vi "UI Visible.vi"(8 "error in (no error)":errorcluster, 10 "UI visible?":bool, 11 "BluePlotHandle in":refnum<class "BluePlotHandle.lvclass">) -> (0 "error out":errorcluster, 3 "BluePlotHandle out":refnum<class "BluePlotHandle.lvclass">)   [LabVIEW 2021, in "BluePlot.lvlib" / "BluePlotHandle.lvclass"]
doc: "This is used to communicate to a plot instance whether or not it is visible.\n\nIf a plot instance is not visible, then it will not update to save performance.\n\nThis is necessary because the plot instance is not able to discern this information by itself"
uses:
  BluePlotHandle.lvclass
  BluePlotHandle.lvclass/BluePlotHandle.ctl
  TypeDefs/plot handle queue data.ctl
  TypeDefs/Plot QSM action.ctl
  BluePlot.lvlib
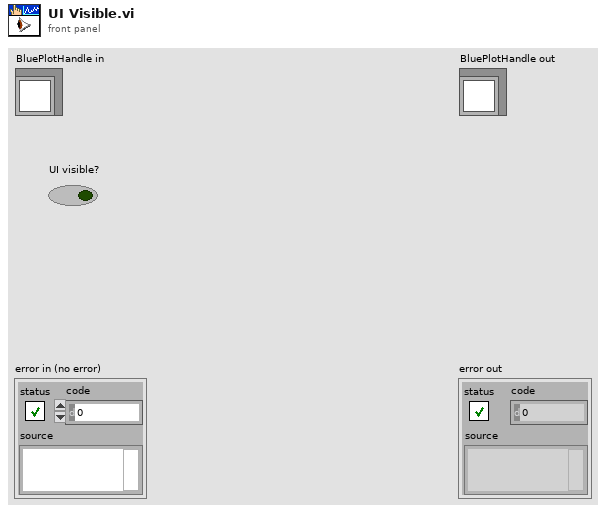
[diagram p1: front panel]
types:
  T1 = typedef "BluePlot.lvlib/Plot QSM action.ctl" = enum16{"start updating", "stop updating", "Shutdown", "Update", "Init", "Get Config", "Load Config"}
  T2 = typedef "BluePlot.lvlib/plot handle queue data.ctl" = cluster{"action":T1, "data":variant}
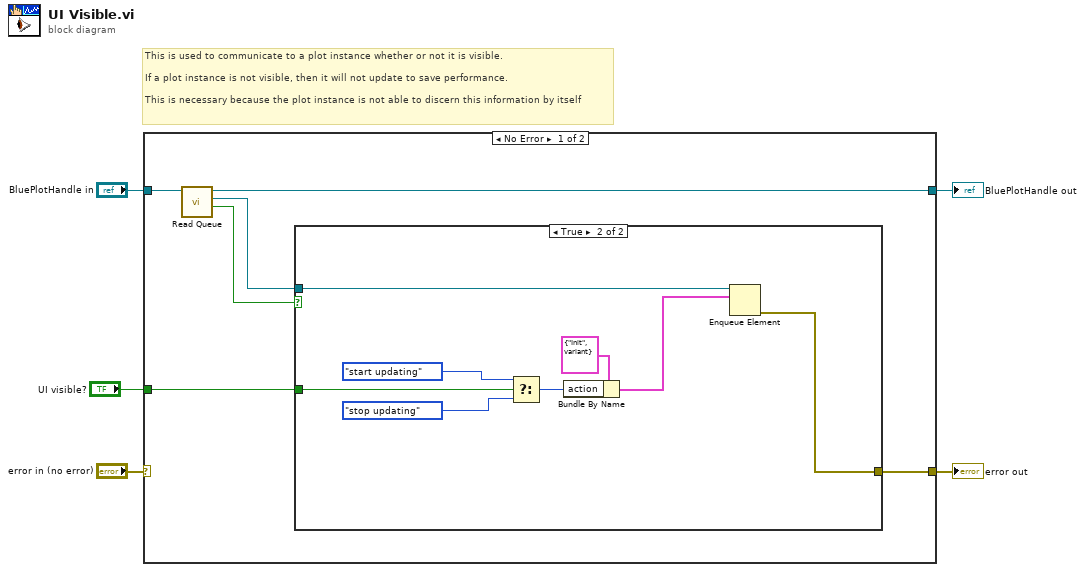
[diagram p0: block diagram]
diagram:
  # "This is used to communicate to a plot instance whether or not it is visible.\n\nIf a plot instance is not visible, then it will not update to save performance.\n\nThis is necessary because the plot instance is not able to discern this information by itself"
  n1 = case shown="No Error" "error in (no error)" {
    selector: "error in (no error)" -> [_ w21]
    tunnel: "BluePlotHandle in" -> [w10 w20]
    tunnel: [w7 w21] -> w3
    tunnel: [w8 w20] -> w4
    tunnel: "UI visible?" -> [w6 _]
    frame No Error {
      n2 = call "Read Queue.vi"("BluePlotHandle in"=w10) -> ("Valid?"=w11:bool, "Queue"=w9:refnum<queue>, "BluePlotHandle out"=w8:refnum<class "BluePlotHandle.lvclass">)  [unwired: 8 in]
      n3 = case shown="True" w11 {
        tunnel: w9 -> [_ w19]
        tunnel: [_ w16] -> w7
        tunnel: w6 -> [_ w15]
        frame False {
        }
        frame True {
          n4 = Select(t=Plot_QSM_action."start updating" ("action"), s=w15, f=Plot_QSM_action."stop updating" ("action")) -> (s? t:f=w13:T1)
          n5 = Bundle By Name(cluster=T2 {"action"=enum."Init", "data"=variant} ("element"), "action"=w13) -> (w17:T2)
          n6 = Enqueue Element(queue=w19, element=w17) -> (error out=w16:errorcluster)  [unwired: 2 in, 2 out]
        }
      }
    }
    frame Error {
    }
  }
  "error out" <- w3
  "BluePlotHandle out" <- w4
